vi "RemoteDmmSession_CallCloseMeasurementLinkSessionWithCloseBehavior_RemoteSessionClosed.vi"(8 "error in":errorcluster) -> (0 "error out":errorcluster, 2 "result":string, 3 "pass":bool)   [LabVIEW 2020, in "MeasurementServerTests.lvlib"]
uses:
  MeasurementServerTests.lvlib
  Runtime/MeasurementLink niDMM/Instrument/Instrument.lvclass
  Runtime/MeasurementLink Instrument/IInstrument/Close Session Behavior.ctl
  Runtime/MeasurementLink Instrument/IInstrument/IInstrument.lvclass
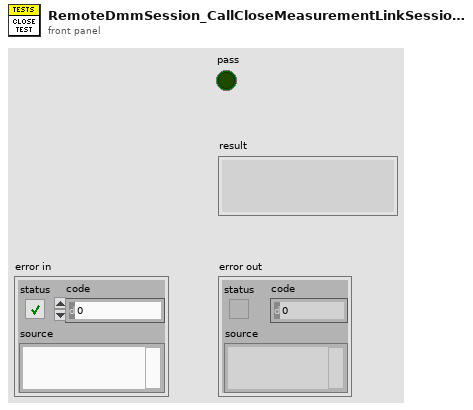
[diagram p1: front panel]
types:
  T1 = typedef "MeasurementLink Instrument.lvlib/IInstrument.lvclass/Remote Connection Options.ctl" = cluster{"session name":string, "address":string, "port":u32}
  T2 = typedef "MeasurementLink Instrument.lvlib/IInstrument.lvclass/Close Session Behavior.ctl" = enum16{"Close Session", "Detach Session"}
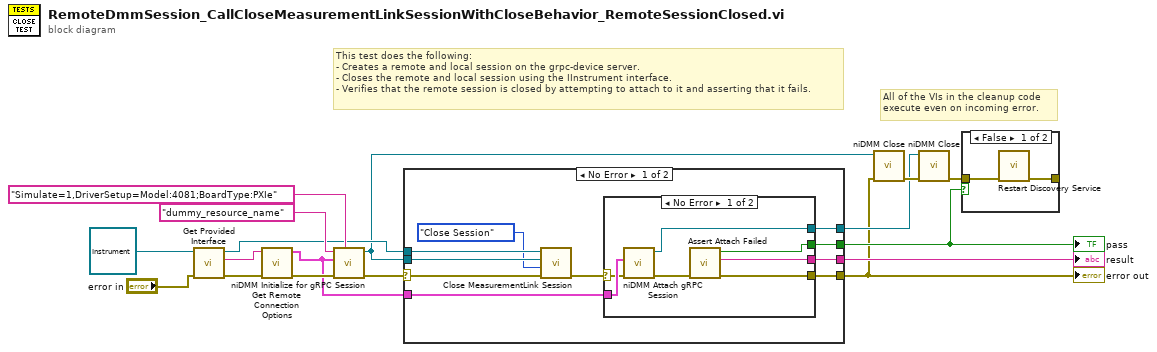
[diagram p0: block diagram]
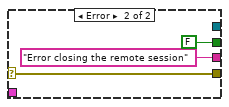
[diagram p2: hidden frame]
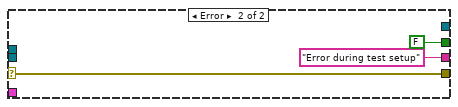
[diagram p3: hidden frame]
diagram:
  # "All of the VIs in the cleanup code\nexecute even on incoming error."
  # "This test does the following:\n- Creates a remote and local session on the grpc-device server.\n- Closes the remote and local session using the IInstrument interface.\n- Verifies that the remote session is closed by attempting to attach to it and asserting that it fails."
  n1 = call-dynamic "Get Provided Interface.vi"("error in"="error in", "instrument in"=refnum<class "Instrument.lvclass"> refnum ("MeasurementLink niDMM.lvlib:Instrument.lvclass")) -> ("error out"=w15:errorcluster, "provided interface"=w14:string, "instrument out"=w11:refnum<class "Instrument.lvclass">)  [unwired: 7 in]
  n2 = call "Get Remote Connection Options.vi"("error in"=w15, "provided interface"=w14) -> ("error out"=w16:errorcluster, "remote connection options"=w10:T1)  [unwired: 8 in]
  n3 = call <instrlib>:"niDMM Initialize for gRPC Session.vi"("Option String"="Simulate=1,DriverSetup=Model:4081;BoardType:PXIe" ("option string"), "error in (no error)"=w16, "gRPC Options"=w10, "Instrument Descriptor"="dummy_resource_name" ("resource name")) -> ("error out"=w12:errorcluster, "instrument handle out"=w6:refnum<k15>)  [unwired: 6 in]
  n4 = case shown="No Error" w12 {
    selector: w12 -> [w27 w39]
    tunnel: w11 -> [w26 _]
    tunnel: w6 -> [w25 _]
    tunnel: w10 -> [w24 _]
    tunnel: [w22 w39] -> w2
    tunnel: [w21 FALSE] -> w7
    tunnel: [w20 "Error during test setup" ("f")] -> w8
    tunnel: [w18 _] -> w4
    frame No Error {
      n5 = call-dynamic "Close MeasurementLink Session.vi"("error in"=w27, "close session behavior"=Close_Session_Behavior."Close Session", "session in"=w25, "instrument in"=w26) -> ("error out"=w23:errorcluster)  [unwired: 7 in]
      n6 = case shown="No Error" w23 {
        selector: w23 -> [w33 w35]
        tunnel: w24 -> [w34 _]
        tunnel: [w30 w35] -> w22
        tunnel: [w32 FALSE] -> w21
        tunnel: [w29 "Error closing the remote session" ("f")] -> w20
        tunnel: [w28 _] -> w18
        frame No Error {
          n7 = call <instrlib>:"niDMM Attach gRPC Session.vi"("error in (no error)"=w33, "gRPC Options"=w34) -> ("error out"=w31:errorcluster, "instrument handle out"=w28:refnum<k15>)  [unwired: 8 in]
          n8 = call "Assert Attach Failed.vi"("error in"=w31) -> ("error out"=w30:errorcluster, "result"=w29:string, "pass?"=w32:bool)  [unwired: 8 in]
        }
        frame Error {
        }
      }
    }
    frame Error {
    }
  }
  "error out" <- w2
  "pass" <- w7
  "result" <- w8
  n9 = call <instrlib>:"niDMM Close.vi"("error in (no error)"=w2, "instrument handle"=w6) -> ("error out"=w5:errorcluster)  [unwired: 9 in]
  n10 = call <instrlib>:"niDMM Close.vi"("error in (no error)"=w5, "instrument handle"=w4) -> ("error out"=w3:errorcluster)  [unwired: 9 in]
  n11 = case shown="False" w7 {
    tunnel: [w42 _] -> _
    tunnel: w3 -> [w41 _]
    frame False {
      n12 = call "Restart Discovery Service.vi"("error in"=w41) -> ("error out"=w42:errorcluster)  [unwired: 10 in]
    }
    frame True {
    }
  }
